vi "Sim_Read_Spectra.vi"(1 "Pixels (512)":i32=512) -> (0 "Array":dbl[](array[numeric])=[0.18522036377910522, 0.6761547591384792, 0.9255514508213534, 0.09331850252571519, 0.899154200339068, 0.6827959176798157, 0.20443579540823537, 0.35221483013466814, 0.7570183601091485, 0.8032852346341256, 0.8257603776992752, 0.8628257014130447, 0.8662593278263044, 0.3015623514352741, 0.3174829013906504, 0.3470443510353399, 0.2707742997614916, 0.8485408075176872, 0.5675687806557213, 0.5750844403881283, 0.8774712605529195, 0.9190509222787386, 0.787564420189085, 0.45809323435313065, 0.6355437092540552, 0.4463106414560434, 0.46356456564431403, 1.1605667611031774, 0.8147978334277487, 1.0685712868922628, 0.7212996297966922, 1.091870856716526, 1.0368330384928868, 1.1066483594426382, 0.42167729857649405, 0.812703715824027, 0.26212940917593114, 1.0405840721339696, 0.37097853835008127, 0.8225837337970207, 0.6464132726499412, 1.217936532700898, 1.2407801475231914, 0.9638622296977929, 0.5545073289300202, 0.6669301113680014, 0.48546667776774916, 1.0920640629332419, 0.7865996792435144, 0.8169229435624914, 1.024724146112556, 0.4950406072634674, 1.1801731328019698, 1.1688234992494728, 1.3184853674496695, 0.6264615022466582, 1.158022943504601, 0.6830532698311782, 1.2347946526241511, 1.0198960235124113, 0.7361174549569613, 0.9293679389410961, 0.729502637889843, 0.8574304682833576, 0.8397814819256924, 1.3282711527544484, 1.0838904393579691, 1.0854398182251306, 1.2954044015045951, 0.41157364731255547, 0.858443625854654, 1.0161136626305365, 0.47096357070854744, 1.3283998307959224, 1.1153259420663604, 1.215448247707529, 1.0872085961779296, 1.0185242022307017, 1.3593576383899282, 0.5635861427213618, 0.6578394371787348, 1.1560273203073557, 1.0344816774305878, 0.635526939892247, 1.3362920187596243, 0.6979817681164842, 0.9606821843661956, 0.9080797156974125, 1.4540599811111758, 1.4492721667138921, 0.9718975630875722, 1.1089850161059576, 1.227905970980105, 1.2419316343896893, 0.7794055495276297, 1.087851429687747, 1.1183704952462257, 1.3161874247253833, 0.9997442359790005, 0.6247070985374062, 0.7231369650156612, 1.0620773102080625, 0.6948984558984002, 1.3911182844579129, 1.1465143249557175, 0.8157750203951369, 1.3709655904268763, 0.8950520587153067, 0.7595162133494202, 1.4782677490967597, 0.9027744118858247, 1.3495025047803253, 0.6380836513541408, 0.8623834569854143, 1.5113659469477796, 1.1309562177157508, 1.5385260551652924, 0.9635188578690165, 0.8116356324359275, 1.4631241658510736, 1.112681622765015, 1.6608171388471025, 0.8404557361088465, 1.6378519513631764, 0.893859509946086, 1.0107000168015428, 0.9247932014418687, 1.4249170879676138, 1.4797678233322413, 0.7676978326879593, 0.8056098537852977, 1.6248192782655324, 1.612174578443104, 1.3362624106352277, 1.3654731263022448, 1.3502329964314774, 1.430189565857449, 0.8234037120200123, 1.3794030607179044, 1.2487920362979417, 1.3029149368321256, 1.0890664682685625, 1.2045345345403775, 1.3644549386777092, 1.3087869508946819, 1.642917012411721, 1.5762953091727725, 1.5243214353438796, 1.3414025085279457, 1.6796147392274552, 1.0509981687135608, 1.172932451352378, 1.7206676757356505, 1.5023669784510818, 1.4739128148214784, 1.4532189334874446, 1.7971220327497237, 1.71768816117505, 1.7028857152014827, 1.6491121328838871, 1.2259522455706953, 1.3055058606788497, 1.6450826336395168, 0.9841488159145261, 1.5054061823935632, 1.6731519080524497, 1.1641546991700542, 0.8821295573689153, 0.9849724538999005, 0.9920039216889902, 1.119005138923428, 0.9901350681006795, 1.0660537551212972, 1.2952551742337142, 1.587682193040909, 1.1797540549298495, 1.7195209535611595, 1.7797578492602713, 1.1587344817392538, 1.8380810752719903, 1.826527047943228, 1.1968589080675947, 1.4387524635960696, 1.7368804263075703, 1.453431207793776, 1.6652978028464394, 1.373396596320796, 1.8806439186920285, 1.734026657638994, 1.5544704316375264, 1.3378497190613683, 1.917985315593472, 1.336470818104305, 1.186592219174583, 0.9321987350105914, 1.3862007596580006, 1.9226347306497236, 1.3627929265212992, 1.7166362493283271, 1.2602719728437333, 1.5026836374423644, 1.1842227527185658, 1.8630941920834982, 1.2368303726967194, 1.8395019061677091, 1.7851573387944144, 1.1983198794635226, 1.1798352372794154, 1.691616034194984, 1.1858699449812589, 1.671815705849701, 1.2430186763035485, 1.0077866762253018, 1.1638169529579336, 1.01113623767164, 1.8103622570038471, 1.7645075373782482, 1.0674314385450767, 1.8550600982890169, 1.165668193769151, 1.7542047739896152, 1.7771038840172522, 1.027418727171212, 1.3364458120640772, 1.6814402766830208, 1.3864553817942382, 1.949505852057106, 1.264331209257971, 1.4629696578935443, 1.4251394273141789, 1.3611701959641531, 1.0365926599797608, 1.1621523906137874, 1.4632330687589068, 1.3249407962084387, 1.6630466682705578, 1.5811137929460308, 1.0119730824584268, 0.9991957943498843, 1.9340860437122105, 1.415266651452518, 1.7234364656650962, 1.8229455340862715, 1.132870422825808, 1.5085222699811554, 1.4112453762643689, 1.602280717117797, 1.5511702475123443, 1.5972301193197929, 1.0580012790747102, 1.9709922738823744, 1.6501893192821946, 1.340132186550787, 1.279920889126734, 1.2933776228589138, 1.3471247043415548, 1.6512342498553423, 1.887324878477873, 1.0458261971215705, 1.2643613719405444, 1.0422697182053406, 1.6105351706695652, 1.7467998343782063, 1.542315745601627, 1.3784667712394447, 1.6947148690503762, 1.9737136229525967, 1.8806087376882092, 1.6136494772961718, 1.1309087739319927, 1.166437649237721, 1.3929221063736767, 1.379422869212316, 1.077008543569148, 1.0696033261842084, 1.55225459204888, 1.5511627056042743, 1.7884984062501834, 1.945965508174059, 1.2189631598172233, 1.8749155384977048, 1.496338215361389, 1.34023842844289, 1.2490964242886475, 1.2209564641090713, 1.5021844695361177, 1.7962741006609224, 1.329571236671554, 1.6202554771881537, 1.22539822750051, 1.4186756748197837, 1.6937157771211329, 1.9519199571486117, 1.24022268766072, 1.2052183145196609, 1.2967852946291711, 1.7507652978865462, 1.6584705034777865, 1.382413258698612, 1.3235093343986444, 1.1209943776208868, 1.5288916675587179, 1.9382740420625477, 1.05301032800459, 1.5254732721299762, 1.7693651354786755, 1.5498300372585225, 1.1068769966460261, 1.1215164687596557, 1.7516015541245087, 1.7350979705073577, 1.6303435152274064, 1.5016675967678244, 1.591645430128501, 1.1928939549255424, 1.4797057134339031, 1.321646302065658, 1.5343457143808057, 1.7954014585400788, 1.3857903118364643, 1.4275518671344987, 1.916920767325439, 1.074245432241847, 1.665978089205604, 1.112579171346653, 1.8653520751107375, 1.1654021164949182, 0.99876927345654, 1.5429119977066994, 1.198026026225246, 1.118028394921554, 1.1749101499489645, 1.0023761734169137, 1.7422163288406947, 0.8906109038071847, 1.1573737692675115, 1.2337649646661317, 1.217492735308515, 1.7493749697527923, 1.7301028548466721, 0.992324671756953, 1.7917216770500737, 1.139930742234674, 1.298938089186444, 1.8137382217866487, 1.5737461617448463, 0.86336796510081, 1.0650960530714737, 1.8361898952030038, 1.4226059468650216, 1.7002380588042623, 1.2522805923295282, 1.609990697569518, 1.0139541104828096, 1.46533794831169, 1.2821328184193463, 0.8893369704956349, 1.5405594371889166, 1.7601254630144991, 1.0408779008080202, 1.0111678703448743, 1.39574672284455, 1.093135778067638, 1.474139512731721, 1.7492588924474586, 1.0581162007111065, 0.9947206517175889, 0.9001182478053193, 1.363663086111609, 1.6191188470049853, 1.216404620863805, 1.3965915840369478, 0.8640289126897996, 1.4322819957095843, 1.3407188647827097, 1.1257301103042674, 0.8638091719584168, 1.5321496285607832, 0.9341766249692575, 1.3578509599623194, 1.69096657308097, 0.9734039976941223, 1.3485948340397709, 1.433524642210251, 1.1192070469724653, 1.2439350935610411, 1.046875194745741, 1.4494240209709006, 0.9321183700170612, 1.0794063988862512, 1.4647061301048039, 0.6881490590867207, 1.587067081326083, 1.2049460864687538, 1.0769845878548086, 1.2299617475912956, 1.0689670806499803, 1.4169320089594508, 1.2113306884094102, 1.114424874948933, 0.9306884387341675, 0.848525936657268, 0.8689885176339833, 0.9681654970182285, 1.1188386381432769, 0.7605447514896919, 0.7525725530690144, 0.7039371742661843, 1.2582695331188136, 0.6299376566838073, 1.3170838324185277, 1.5070476690159658, 1.0701227736588148, 1.1134156283052725, 1.3083395883023716, 1.4232625296609513, 0.6790221870059758, 1.3042415955223534, 1.4379907767489288, 0.7244333184509192, 1.500502592913565, 1.0219948959350704, 0.8013894466237078, 1.1657221508532791, 0.938530083274822, 0.9869143392228474, 1.4631959123615745, 1.0147600247395359, 1.0393801311152617, 0.7566138360051486, 1.34568369554216, 0.920318633951485, 0.883812807842731, 0.5600494988401424, 0.5111366514109861, 1.3303812535377284, 0.5176414168351, 0.6309230825550436, 1.0426919141809474, 0.97633629065961, 0.6137715442604752, 1.4052065270373113, 1.1451563768565478, 1.117752253251347, 0.8717836603539513, 0.8274523176741855, 0.7701539197461651, 1.113861751537372, 1.1174877682135451, 0.8901484183444703, 1.0783218019630838, 0.5022332279717753, 1.1481279987062125, 0.4669642150444114, 0.6931075245806513, 1.0182571457294776, 1.2480940887497887, 1.0128312721425297, 0.3617793512462074, 1.2693952754078968, 0.7386091852129464, 1.1416413066849869, 1.0448273596519704, 0.8237247055132302, 0.9818095805973353, 0.3355503468118014, 0.5414021407383486, 0.3630875535224619, 0.4181967137554483, 1.1135314973962203, 0.31493046725545043, 0.9811345247895811, 0.416943136880794, 0.6701113646511441, 0.38263727503362543, 1.1602325195829495, 0.49640447982944014, 0.23787549130792948, 0.6836084236307431, 0.5698557268063924, 0.41533992510555406, 0.9878355067587958, 0.3709923074840833, 1.0247945289123042, 1.0319933105622043, 0.5226164570972807, 0.3999099248390858, 0.6232453828913451, 0.917334635334526, 0.8524191911775176, 0.39594096926489697, 1.0097503632662743, 0.9176510071573859, 0.6613941376036905, 0.9771804372599184, 1.0328869479542486, 0.6825103080059526, 0.2528829262358322, 0.914445971747301, 0.9359366619657368, 0.7294989498666793, 0.09405208521046535, 0.4913882060702431, 0.14791908345328192, 0.9587901940916246, 0.8720546043484677, 0.0682009342421864, 0.08511354668365062, 0.15711932479437496, 0.3895454073542326, 0.39007428380679465, 0.04874302917196711])   [LabVIEW 2018]
panel:
  out "XY Graph":cluster{"Y":dbl[], "Y":dbl[]}[](graph)
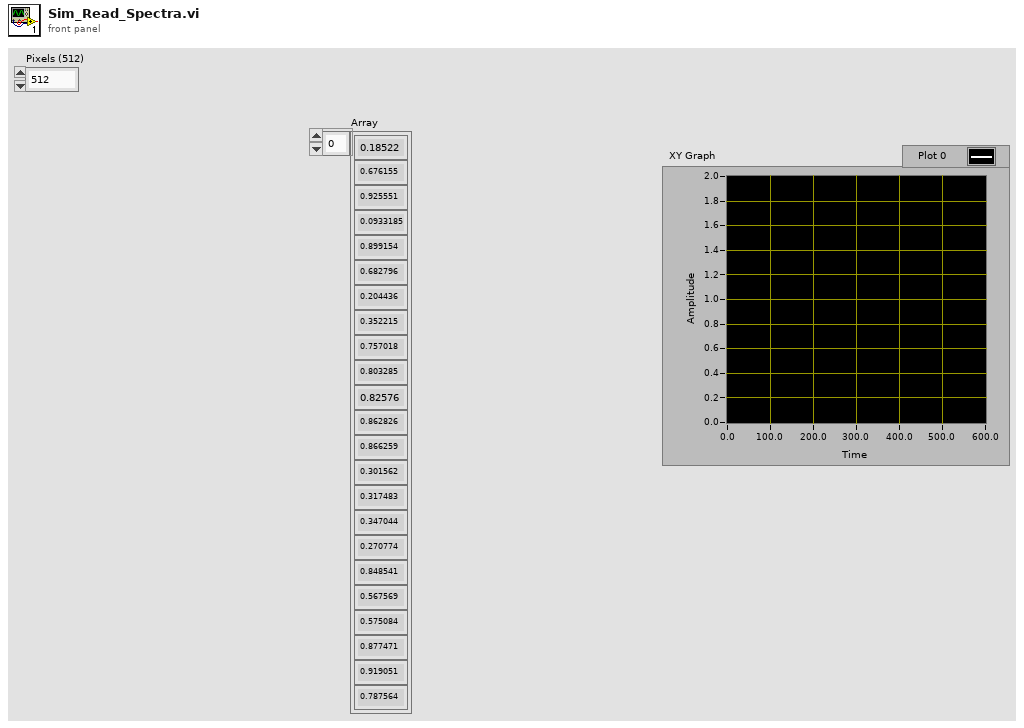
[diagram p1: front panel]
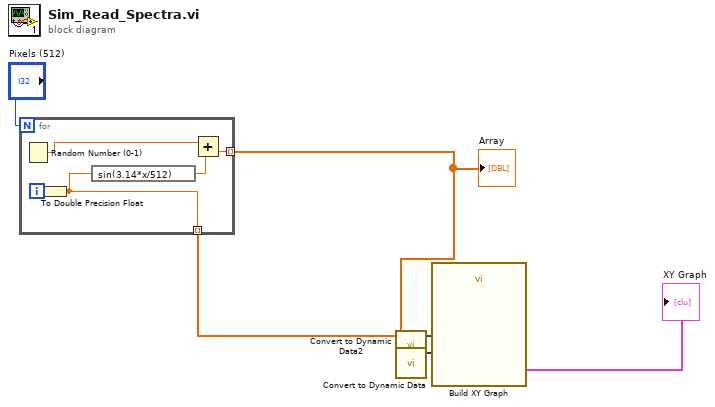
[diagram p0: block diagram]
diagram:
  n1 = for {
    N: "Pixels (512)" -> [_]
    tunnel: [w8] -> w4 mode=indexing
    tunnel: [w9] -> w2 mode=indexing
    i -> [w11]
    n2 = Random Number (0-1)() -> (number: 0 to 1=w7:dbl)
    n3 = To Double Precision Float(number=w11) -> (double precision float=w9:dbl)
    n4 = expression code="sin(3.14*x/512)"(w9) -> (w10:dbl)
    n5 = Add(x=w7, y=w10) -> (x+y=w8:dbl)
  }
  "Array" <- w4
  n6 = call "Convert to Dynamic Data2"("Array"=w2) -> ("Dynamic Data Type"=w1:dynamicdata)  [unwired: 3 in]
  n7 = call "Convert to Dynamic Data"("Array"=w4) -> ("Dynamic Data Type"=w3:dynamicdata)  [unwired: 3 in]
  n8 = call "Build XY Graph"("Y Input"=w3, "X Input"=w1) -> ("XY Graph"=→"XY Graph":cluster{"X":dbl[], "Y":dbl[]}[])  [unwired: 8 in, 1 out]
